vi "XIPIN_Convolution_Encoder_8_0.vi"   [LabVIEW 2017]
doc: "The Convolutional Encoder LogiCORE from Xilinx is a high-speed, compact convolutional encoder with a puncturing option. The Convolutional Encoder core is parameterizable, allowing the designer to control the constraint length and the type of convolutional and puncture code. The core is delivered through the Xilinx CORE Generator System and integrates seamlessly with the Xilinx design flow.\n------------------------------------\n<b>Need License</b> : No\n<b>Interface</b> : AXI4-Stream"
uses:
  <vilib>/rvi/XilinxIP/XIPIN_XNode/niFpgaXIPIN.xnode
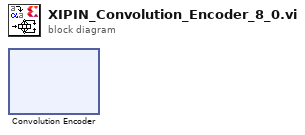
[diagram p0: block diagram]
diagram:
  n1 = xnode ("Convolution Encoder")() -> ()
